vi "Write Buses.vi"(8 "error in (no error)":errorcluster, 10 "Buses":refnum<class "Bus_Access.lvclass">[](array[class]), 11 "Remap Bus in":refnum<class "Remap Bus.lvclass">) -> (0 "error out":errorcluster, 3 "Remap Bus out":refnum<class "Remap Bus.lvclass">)   [LabVIEW 2021, in "Remap Bus.lvclass"]
uses:
  Remap Bus.lvclass
  Omni-Bus/Bus Access/Bus_Access.lvclass
  Remap Bus.lvclass/Remap Bus.ctl
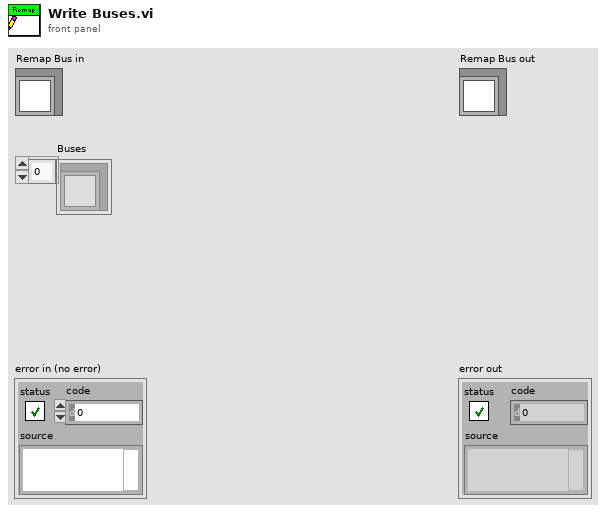
[diagram p1: front panel]
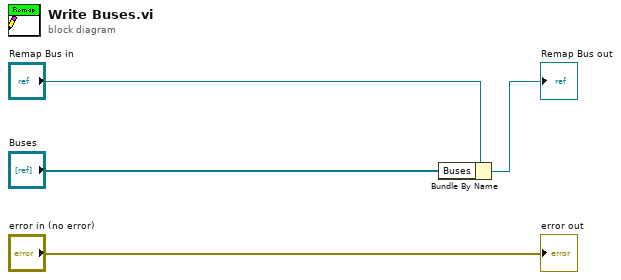
[diagram p0: block diagram]
diagram:
  n1 = Bundle By Name(cluster="Remap Bus in", "Buses"="Buses") -> (→"Remap Bus out":refnum<class "Remap Bus.lvclass">)
  "error out" <- "error in (no error)"
